vi "FGV Komponentenreferenzen verwalten.vi"(0 "Referenzen":refnum<vi>[](array[refnum]), 7 "Strings []":string[](array[string]), 11 "error in (no error)":errorcluster caption="Fehler (Eingang, kein Fehler)", 13 "Aktion":T1) -> (15 "error out":errorcluster caption="Fehler (Ausgang)")   [LabVIEW 2020, in "EPA 1065.lvlib" / "Gas Analyzer Drift 1065-550.lvlib"]
uses:
  Gas Analyzer Drift 1065-550.lvlib
  Aktion FGV Komponentenreferenz verwalten.ctl
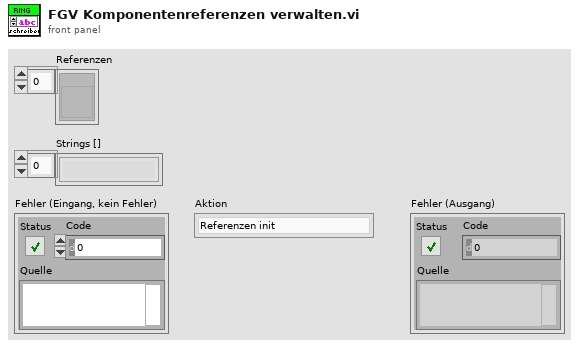
[diagram p1: front panel]
types:
  T1 = typedef "EPA 1065.lvlib/Gas Analyzer Drift 1065-550.lvlib/Aktion FGV Komponentenreferenz verwalten.ctl" = enum16{"Referenzen init", "lesen", "Referenzen schließen", "Ring beschreiben"}
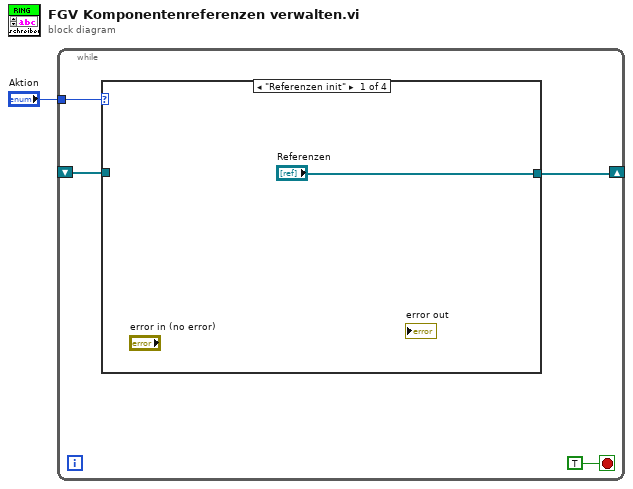
[diagram p0: block diagram]
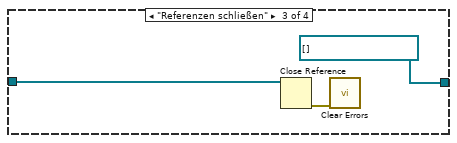
[diagram p3: hidden frame]
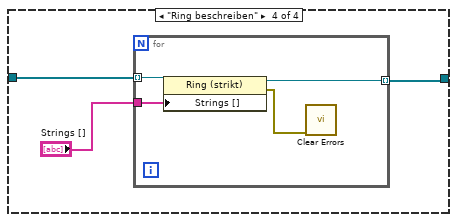
[diagram p4: hidden frame]
diagram:
  n1 = while {
    tunnel: "Aktion" -> [w5]
    shift-right: [w3] -> _
    shift-left: _ -> [w2]
    stop <- TRUE stop-if-true
    n2 = case shown="\"Referenzen init\"" w5 {
      tunnel: ["Referenzen" w7 refnum<vi>[] [] ("Referenzen") w12] -> w3
      tunnel: w2 -> [_ w7 w10 w13]
      frame "Referenzen init" {
      }
      frame "lesen", Default {
      }
      frame "Referenzen schließen" {
        n3 = Close Reference(reference=w10) -> (error out=w8:errorcluster)  [unwired: 1 in]
        n4 = call <vilib>:"Clear Errors.vi"("error in (no error)"=w8) -> ()  [unwired: 5 in, 2 out]
      }
      frame "Ring beschreiben" {
        n5 = for {
          tunnel: w13 -> [w17] mode=indexing
          tunnel: [w16] -> w12 mode=indexing
          tunnel: "Strings []" -> [w14]
          n6 = property on="Eigenschaftsknoten" class="Ring (strikt)"(reference=w17, "Strings []"=w14) -> (reference out=w16:refnum<vi>, error out=w15:errorcluster)  [unwired: 1 in]
          n7 = call <vilib>:"Clear Errors.vi"("error in (no error)"=w15) -> ()  [unwired: 5 in, 2 out]
        }
      }
    }
  }
